vi "FTW-CodeGen-ChooseImplementation.vi"(0 "GObject to Traverse":refnum<vi>, 5 "Diagram Disable Structure Label":string="@FTW-CodeGen", 7 "Frame to Keep":u32, 11 "error in":errorcluster) -> (4 "GObject to Traverse out":refnum<vi>, 15 "error out":errorcluster)   [LabVIEW 2015]
panel:
  # "Inputs"
  # "Outputs"
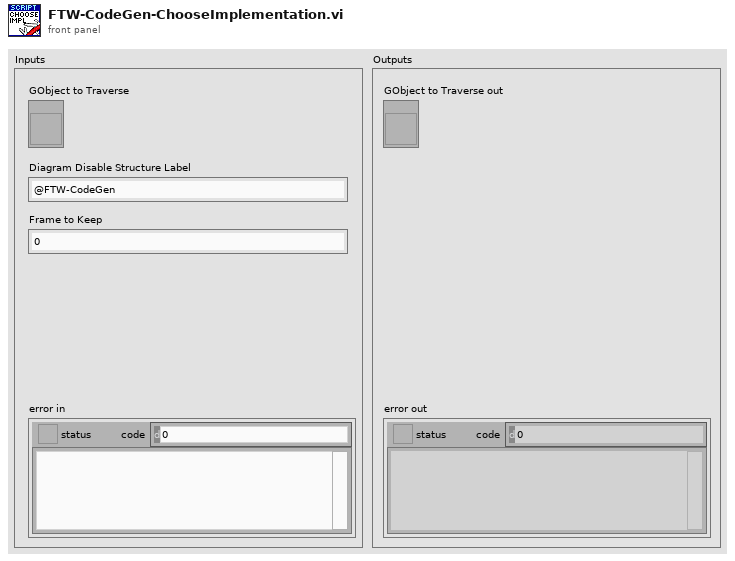
[diagram p1: front panel]
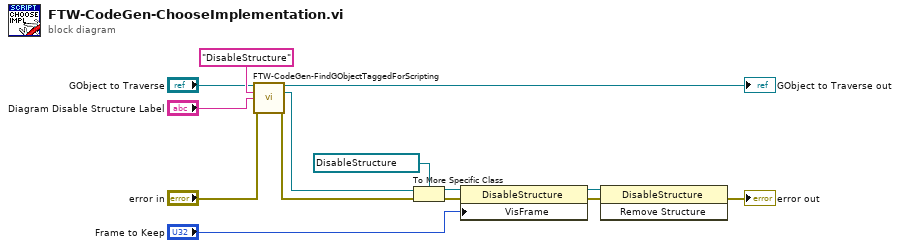
[diagram p0: block diagram]
diagram:
  n1 = call "FTW-CodeGen-FindGObjectTaggedForScripting.vi"("GObject to Traverse"="GObject to Traverse", "Class Name"="DisableStructure", "Label Prefix to uniquely identify node"="Diagram Disable Structure Label", "error in"="error in") -> ("GObject to Traverse out"=→"GObject to Traverse out":refnum<vi>, "GObject"=w13:refnum<vi>, "error out"=w12:errorcluster)  [unwired: 9 in]
  n2 = To More Specific Class(target class=refnum<vi> refnum ("Object"), reference=w13, error in=w12) -> (specific class reference=w11:refnum<vi>, error out=w10:errorcluster)
  n3 = property class="DisableStructure"(reference=w11, error in=w10, "VisFrame"="Frame to Keep") -> (reference out=w5:refnum<vi>, error out=w3:errorcluster)
  n4 = invoke class="DisableStructure" method="Remove Structure"(reference=w5, error in=w3) -> (error out=→"error out":errorcluster)  [unwired: 1 in, 2 out]
